vi "Do Sequence Actions.vi"(9 "Last Sequence Time":i32, 11 "Current Sequence Time":i32) -> (2 "Executed Action Idx":i32)   [LabVIEW 2015]
uses:
  Sequence Global Action.ctl
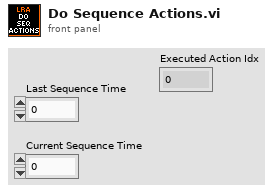
[diagram p1: front panel]
types:
  T1 = typedef "Sequence Global Action.ctl" = enum16{"Get", "Set List", "Set Current"}
  T2 = typedef "Single Test Sequence.ctl" = cluster{"Actions":T3[], "Triggers":T6[], "Name":string}
  T3 = typedef "Test Sequence Action.ctl" = cluster{"Time":i32, "Action":T4, "Valve":T5}
  T4 = typedef "Valve Action Enum.ctl" = enum16{"Open", "Close"}
  T5 = typedef "Valve Name Enum.ctl" = enum16{"FV-2", "FV-3", "FV-4", "OV-2", "OV-3", "OV-4", "NV-2", "COMP"}
  T6 = typedef "Test Sequence Trigger.ctl" = cluster{"Sensor":T7, "Begin Time (ms)":u32, "End Time(ms)":u32, "Min Value":dbl, "Max Value":dbl, "Exceed Action":string}
  T7 = typedef "Sensor Enum.ctl" = enum16{"FPD-1", "FPD-2", "FPD-3", "OPD-1", "OPD-2", "OPD-3", "AP-1", "PC-1", "PC-2", "VBAT", "VCOMP", "ICOMP", "TC-1", "TC-COMP"}
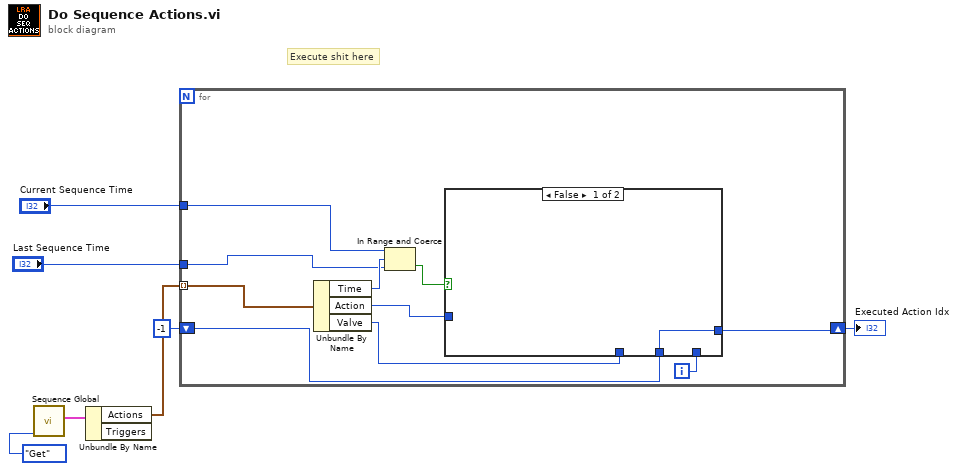
[diagram p0: block diagram]
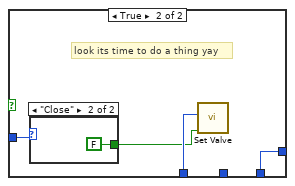
[diagram p2: hidden frame]
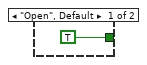
[diagram p3: hidden frame]
diagram:
  # "Execute shit here"
  n1 = call "Sequence Global.vi"("Action"=Sequence_Global_Action."Get") -> ("Current Sequence"=w6:T2)  [unwired: 8 in, 2 out]
  n2 = Unbundle By Name(w6) -> ("Actions"=w7:T3[])  [unwired: 1 out]
  n3 = for {
    tunnel: w7 -> [w17] mode=indexing
    tunnel: "Last Sequence Time" -> [w12]
    tunnel: "Current Sequence Time" -> [w11]
    shift-right: [w9] -> w1
    shift-left: -1 -> [w8]
    i -> [w10]
    n4 = Unbundle By Name(w17) -> ("Time"=w16:i32, "Action"=w14:T4, "Valve"=w13:T5)
    n5 = In Range and Coerce(upper limit=w11, x=w16, lower limit=w12) -> (In Range?=w15:bool)  [unwired: 1 out]
    n6 = case shown="False" w15 {
      tunnel: w14 -> [_ w22]
      tunnel: w13 -> [_ w21]
      tunnel: [w18 w19] -> w9
      tunnel: w10 -> [_ w19]
      tunnel: w8 -> [w18 _]
      frame False {
      }
      frame True {
        # "look its time to do a thing yay"
        n7 = case shown="\"Close\"" w22 {
          tunnel: [TRUE FALSE] -> w20
          frame "Open", Default {
          }
          frame "Close" {
          }
        }
        n8 = call "Set Valve.vi"("New State"=w20, "Valve"=w21) -> ()  [unwired: 10 in]
      }
    }
  }
  "Executed Action Idx" <- w1
